vi "数组元素拼接成字符串.vi"(1 "输入数组":dbl[](array[numeric])) -> (0 "输出字符串":string)   [LabVIEW 2019]
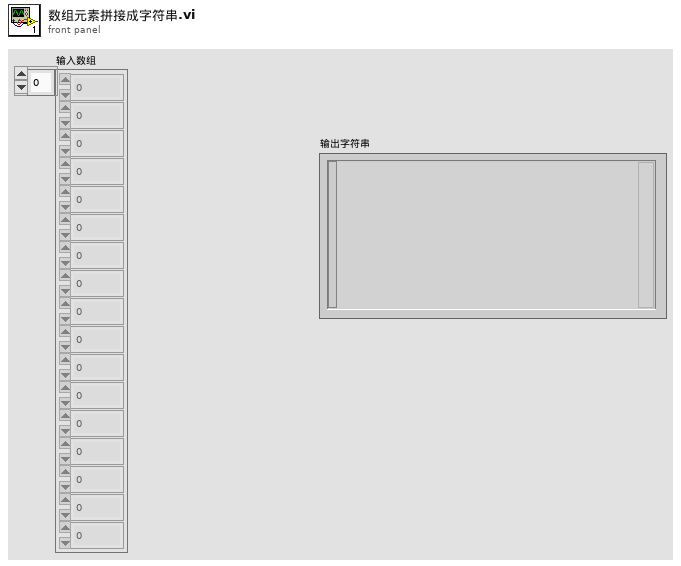
[diagram p1: front panel]
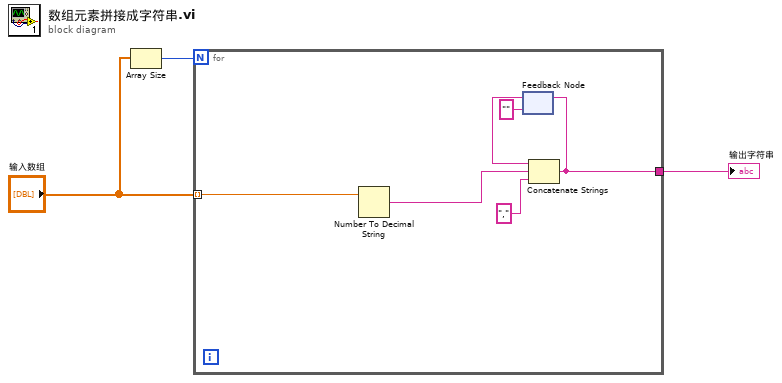
[diagram p0: block diagram]
diagram:
  n1 = Array Size(array="输入数组") -> (size(s)=w2:i32)
  n2 = for {
    N: w2 -> [_]
    tunnel: "输入数组" -> [w9] mode=indexing
    tunnel: [w5] -> w1
    n3 = Number To Decimal String(number=w9) -> (decimal integer string=w7:string)  [unwired: 1 in]
    n4 = feedback #1("") -> (w8:string)
    n5 = Concatenate Strings(w8, w7, "," ("字符串")) -> (w5:string)
    n6 = feedback-in #1(w5) -> ()
  }
  "输出字符串" <- w1
